vi "7_Hole_Probe Pressures to UVW_All_Ps.vi"() -> ()   [LabVIEW 2017]
uses:
  Controls/Setup.ctl
  Globals/Meas_global.vi
panel:
  in  "Desired Freq Hz":dbl=50.0
  out "Averaging samples":i32=5
  out "Current Case":string
  out "UVW chs":i32[](array[numeric])
  out "UVW":dbl[][](array[numeric])
  out "7 Hole Probe chs":string[](array[string])
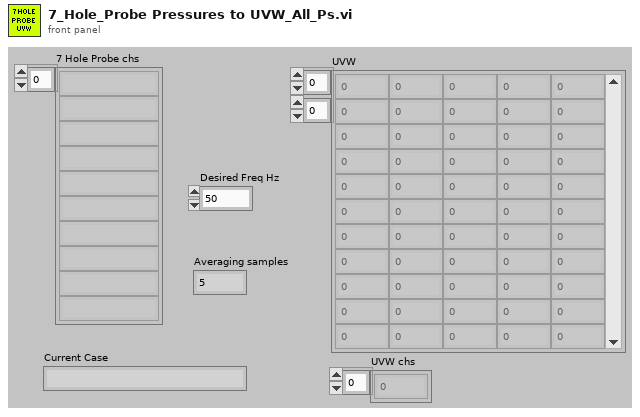
[diagram p1: front panel]
types:
  T1 = typedef "Analysis_info_cluster.ctl" = cluster{"Colour":u32, "Inst type":T2, "Inst name":string, "Symbol":string, "Code name":string, "Extra Info":string, "Inst Array":T3, "Extra Titles":string[], "Extra Values":string[], "U":dbl, "u^2":dbl, "u^3":dbl, "u^4":dbl, "Skew_u":dbl, "Kurt_u":dbl, "Sd Error in Mean":dbl, "% u'/U":dbl, "X":dbl, "Y":dbl, "Z":dbl, "Timescale integral Estimate":dbl, "Sd Error in Variance":dbl, "Calib File":path, "Calib Constants":dbl[], "Output Position":bool, "Full Stats":bool, "Av Sampling Rate":dbl, "Av No of Samples":dbl, "Total Meas Time (s)":dbl, "ADAM Ch Name":string, "Max value":dbl, "Min value":dbl, "Req Sample Rate Hz":dbl, "Sync Delay Time (s)":dbl, "Ch No":i16, "Device ID":string, "Use Latest Calib":bool, "Port":string}
  T2 = typedef "Inst_type.ctl" = enum16{"Propeller anemometer", "Raw voltage", "Pressure Transducer", "Pitot-static tube", "Preston tube", "Hot wire", "Cross wire 1", "Cross wire 2", "Generic Linear", "Generic Polynomial", "Generic BackPoly", "Fast FID", "Thermocouple", "Cold wire", "Pulsed Wire", "LDA Vel", "LDA Tran time", "LDA Arr time", "Microphone"}
  T3 = typedef "Instrument_Array.ctl" = enum16{"PWA", "LDA", "Analogue"}
  T4 = typedef "Time_Trace_Cluster.ctl" = cluster{"Weighting":dbl[], "Time (s)":dbl[], "Voltage":dbl[], "Eng Values":dbl[]}
  T5 = typedef "Setup.ctl" = enum16{"Run Program", "Show Setup", "Save Current Setup", "Setup Front Panel"}
  T6 = cluster{"Pressure Ch Names":string[], "Pressure Index":i32[], "Metadata Index":i32[], "Port":string}[]
  T7 = cluster{"Pressure Ch Names":string[], "Pressure Index":i32[], "Metadata Index":i32[], "Port":string}
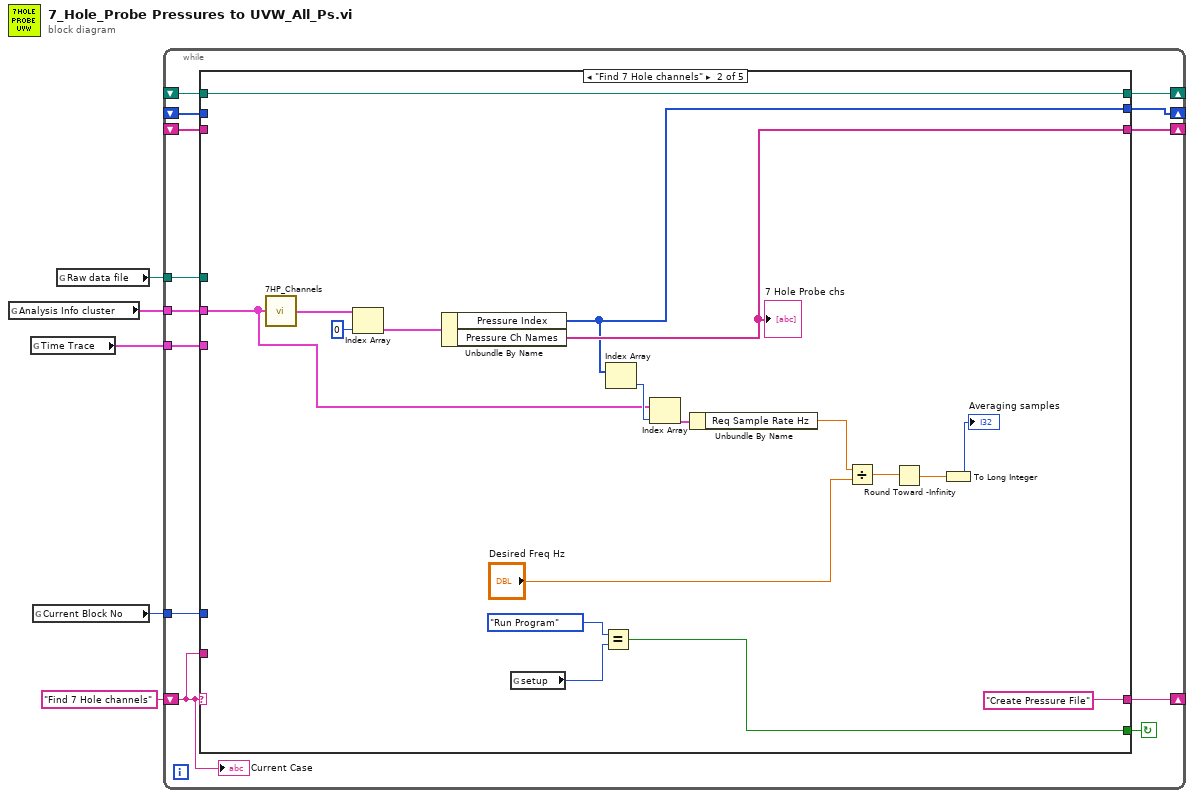
[diagram p0: block diagram]
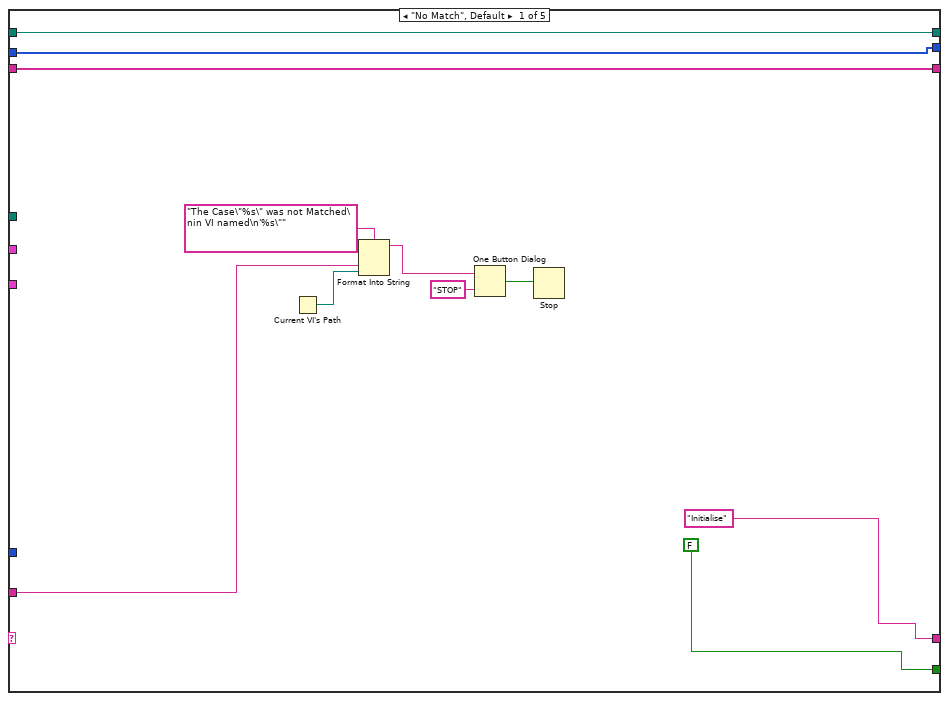
[diagram p2: hidden frame]
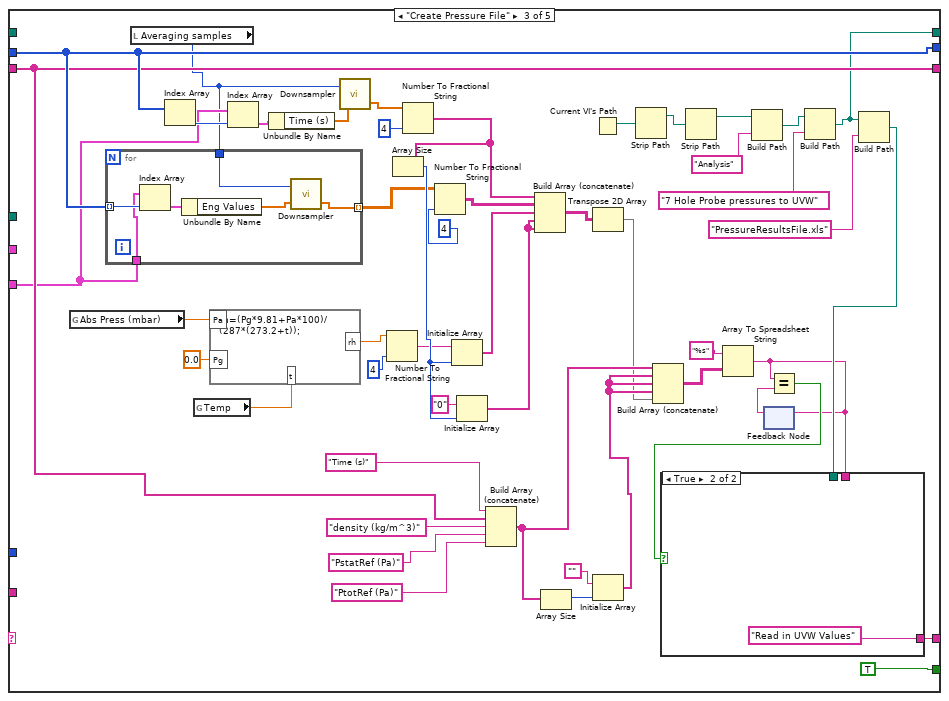
[diagram p3: hidden frame]
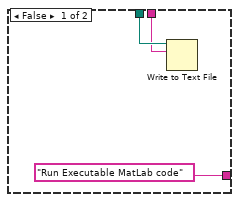
[diagram p4: hidden frame]
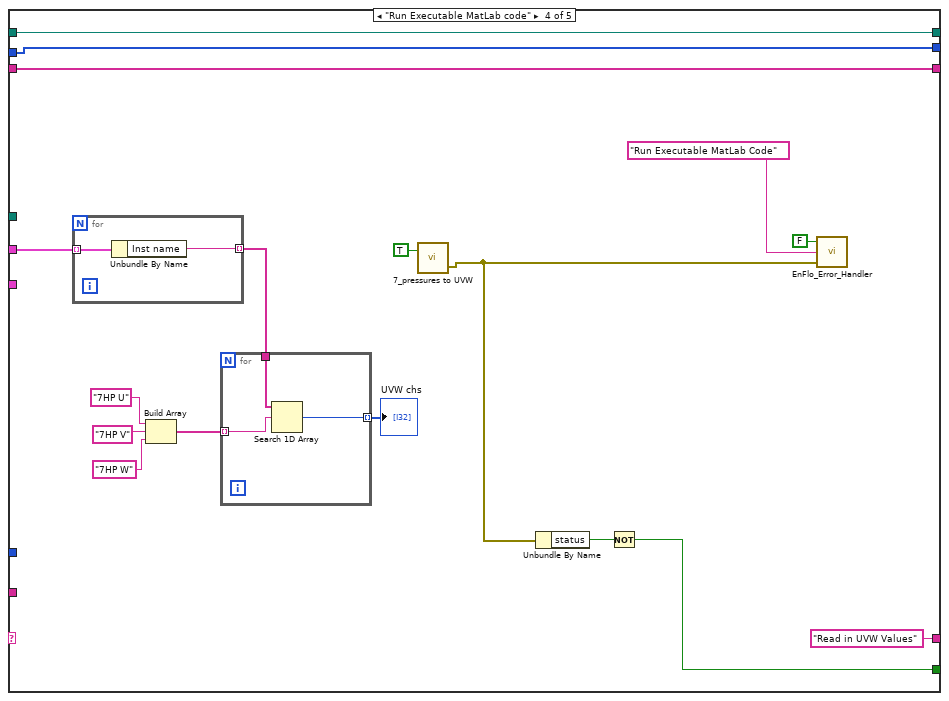
[diagram p5: hidden frame]
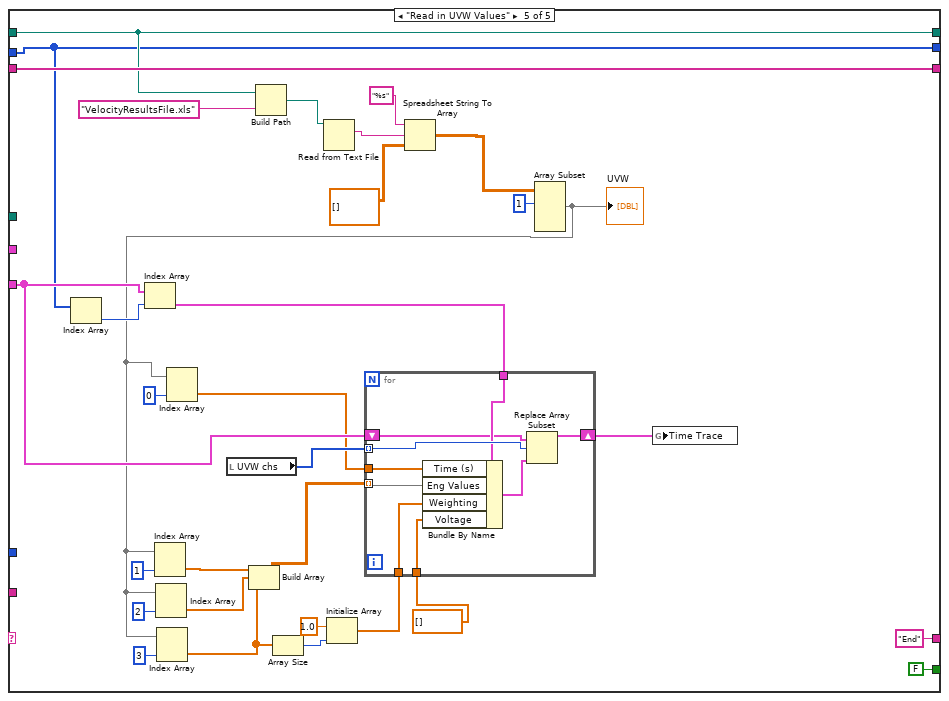
[diagram p6: hidden frame]
diagram:
  n1 = global read "Meas_global.vi" "Analysis Info cluster"() -> (w3:T1[])
  n2 = global read "Meas_global.vi" "Time Trace"() -> (w2:T4[])
  n3 = global read "Meas_global.vi" "Current Block No"() -> (w1:i32)
  n4 = global read "Meas_global.vi" "Raw data file"() -> (w4:path)
  n5 = while {
    shift-left: "Find 7 Hole channels" -> [w6]
    shift-right: [w7] -> _
    tunnel: w4 -> [w17]
    tunnel: w3 -> [w16]
    shift-right: [w15] -> _
    shift-left: _ -> [w14]
    shift-right: [w13] -> _
    shift-left: _ -> [w12]
    shift-right: [w11] -> _
    shift-left: _ -> [w10]
    tunnel: w2 -> [w9]
    tunnel: w1 -> [w8]
    stop <- w18 continue-if-true
    n6 = case shown="\"Find 7 Hole channels\"" w6 {
      tunnel: [FALSE w43 TRUE w107 FALSE] -> w18
      tunnel: ["Initialise" "Create Pressure File" ("t") w95 "Read in UVW Values" ("t") "End" ("t")] -> w7
      tunnel: w6 -> [w24 _ _ _ _]
      tunnel: w17 -> [_ _ _ _ _]
      tunnel: w16 -> [_ w36 _ w115 _]
      tunnel: [w21 w38 w94 w123 w139] -> w15
      tunnel: w14 -> [w21 _ w94 w123 w139]
      tunnel: [w20 w39 w69 w122 w159] -> w13
      tunnel: w12 -> [w20 _ w69 w122 w159]
      tunnel: [w19 w46 w55 w111 w156] -> w11
      tunnel: w10 -> [w19 w46 _ w111 w156]
      tunnel: w9 -> [_ _ w54 _ w140]
      tunnel: w8 -> [_ _ _ _ _]
      frame "No Match", Default {
        n7 = Current VI's Path() -> (path=w23:path)
        n8 = Format Into String(format string="The Case\"%s\" was not Matched\nin VI named\n'%s\"" ("Format String"), w24, w23) -> (resulting string=w27:string)  [unwired: 2 in, 1 out]
        n9 = One Button Dialog(message=w27, button name ("OK")="STOP") -> (true=w25:bool)
        n10 = Stop(stop? (T)=w25) -> ()
      }
      frame "Find 7 Hole channels" {
        n11 = call "7HP_Channels.vi"("Analysis Info cluster"=w36) -> ("7HP Info"=w42:T6)
        n12 = Index Array(array=w42, index=0 ("index (row)")) -> (element=w40:T7)
        n13 = Unbundle By Name(w40) -> ("Pressure Index"=w38:i32[], "Pressure Ch Names"=w39:string[])
        "7 Hole Probe chs" <- w39
        n14 = global read "Meas_global.vi" "setup"() -> (w45:T5)
        n15 = Equal?(x=Setup."Run Program" ("setup"), y=w45) -> (x = y?=w43:bool)
        n16 = Index Array(array=w38) -> (element=w37:i32)  [unwired: 1 in]
        n17 = Index Array(array=w36, index=w37) -> (element=w35:T1)
        n18 = Unbundle By Name(w35) -> ("Req Sample Rate Hz"=w34:dbl)
        n19 = Divide(x=w34, y="Desired Freq Hz") -> (x/y=w32:dbl)
        n20 = Round Toward -Infinity(1:w32) -> (0:w31:dbl)
        n21 = To Long Integer(number=w31) -> (32bit integer=→"Averaging samples":i32)
      }
      frame "Create Pressure File" {
        n22 = global read "Meas_global.vi" "Abs Press (mbar)"() -> (w90:dbl)
        n23 = local read "Averaging samples"() -> (w48:i32)
        n24 = for {
          tunnel: w94 -> [w106] mode=indexing
          tunnel: [w102] -> w77 mode=indexing
          tunnel: w54 -> [w104]
          tunnel: w48 -> [w101]
          n25 = Index Array(array=w104, index=w106) -> (element=w105:T4)
          n26 = Unbundle By Name(w105) -> ("Eng Values"=w103:dbl[])
          n27 = call "Downsampler.vi"("Input Array"=w103, "Averaging samples"=w101) -> ("Downsampled Array"=w102:dbl[])  [unwired: 1 out]
        }
        n28 = Index Array(array=w94) -> (element=w92:i32)  [unwired: 1 in]
        n29 = global read "Meas_global.vi" "Temp"() -> (w91:dbl)
        n30 = formula code="rh=(Pg*9.81+Pa*100)/\n(287*(273.2+t));"("t"=w91, "Pg"=0.0 ("input variable"), "Pa"=w90) -> ("rh"=w74:dbl)
        n31 = Index Array(array=w54, index=w92) -> (element=w93:T4)
        n32 = Unbundle By Name(w93) -> ("Time (s)"=w50:dbl[])
        n33 = call "Downsampler.vi"("Input Array"=w50, "Averaging samples"=w48) -> ("Downsampled Array"=w49:dbl[])  [unwired: 1 out]
        n34 = Number To Fractional String(number=w74, precision (6)=i16 4) -> (F-format string=w73:string)  [unwired: 2 in]
        n35 = Number To Fractional String(number=w49, precision (6)=i16 4) -> (F-format string=w79:string[])  [unwired: 2 in]
        n36 = Array Size(array=w79) -> (size(s)=w88:i32)
        n37 = Number To Fractional String(number=w77, precision (6)=i16 4) -> (F-format string=w76:string[][])  [unwired: 2 in]
        n38 = Initialize Array(w73, w88) -> (w86:string[])
        n39 = Initialize Array("0" ("element"), w88) -> (w85:string[])
        n40 = Build Array (concatenate)("Time (s)", w69, "density (kg/m^3)", "PstatRef (Pa)", "PtotRef (Pa)") -> (w60:string[])
        n41 = Build Array (concatenate)(w79, w76, w86, w85, w85) -> (w72:string[][])
        n42 = Array Size(array=w60) -> (size(s)=w59:i32)
        n43 = Current VI's Path() -> (path=w68:path)
        n44 = Transpose 2D Array(2D array=w72) -> (transposed array=w56:string[][])
        n45 = Initialize Array("", w59) -> (w57:string[])
        n46 = Strip Path(path=w68) -> (stripped path=w67:path)  [unwired: 1 out]
        n47 = Build Array (concatenate)(w60, w57, w57, w57, w56) -> (w71:string[][])
        n48 = Strip Path(path=w67) -> (stripped path=w66:path)  [unwired: 1 out]
        n49 = Array To Spreadsheet String(array=w71, 3:"%s" ("format string")) -> (spreadsheet string=w51:string)  [unwired: 1 in]
        n50 = Build Path(base path=w66, name or relative path="Analysis") -> (appended path=w64:path)
        n51 = feedback-in #1(w51) -> ()
        n52 = feedback #1() -> (w53:string)  [unwired: 1 in]
        n53 = Equal?(x=w51, y=w53) -> (x = y?=w52:bool)
        n54 = Build Path(base path=w64, name or relative path="7 Hole Probe pressures to UVW") -> (appended path=w55:path)
        n55 = Build Path(base path=w55, name or relative path="PressureResultsFile.xls") -> (appended path=w61:path)
        n56 = case shown="True" w52 {
          tunnel: ["Run Executable MatLab code" ("t") "Read in UVW Values" ("t")] -> w95
          tunnel: w61 -> [w99 _]
          tunnel: w51 -> [w98 _]
          frame False {
            n57 = Write to Text File(file (use dialog)=w99, text=w98) -> ()  [unwired: 2 in, 3 out]
          }
          frame True {
          }
        }
      }
      frame "Run Executable MatLab code" {
        n58 = for {
          tunnel: w115 -> [w128] mode=indexing
          tunnel: [w127] -> w114 mode=indexing
          n59 = Unbundle By Name(w128) -> ("Inst name"=w127:string)
        }
        n60 = Build Array("7HP U" ("Inst name"), "7HP V" ("Inst name"), "7HP W" ("Inst name")) -> (w113:string[])
        n61 = for {
          tunnel: w114 -> [w126]
          tunnel: w113 -> [w125] mode=indexing
          tunnel: [w124] -> w112 mode=indexing
          n62 = Search 1D Array(1D array=w126, element=w125) -> (index of element=w124:i32)  [unwired: 1 in]
        }
        "UVW chs" <- w112
        n63 = call "7_pressures to UVW.vi"("wait until completion?"=TRUE) -> ("error out"=w109:errorcluster)  [unwired: 2 in]
        n64 = Unbundle By Name(w109) -> ("status"=w108:bool)
        n65 = Not(x=w108) -> (.not. x?=w107:bool)
        n66 = call "EnFlo_Error_Handler.vi"("error in (no error)"=w109, "Error Type"="Run Executable MatLab Code", "Dialog Box (T)"=FALSE) -> ()  [unwired: 3 out]
      }
      frame "Read in UVW Values" {
        n67 = Index Array(array=w139) -> (element=w138:i32)  [unwired: 1 in]
        n68 = Index Array(array=w140, index=w138) -> (element=w137:T4)
        n69 = local read "UVW chs"() -> (w141:i32[])
        n70 = Build Path(base path=w156, name or relative path="VelocityResultsFile.xls") -> (appended path=w154:path)
        n71 = Read from Text File(file (use dialog)=w154) -> (text=w153:string)  [unwired: 3 in, 3 out]
        n72 = Spreadsheet String To Array(format string="%s", spreadsheet string=w153, array type (2D Dbl)=dbl[][] []) -> (array=w150:dbl[][])  [unwired: 1 in]
        n73 = Array Subset(array=w150, index (row)=1 ("index")) -> (w135:dbl[][])  [unwired: 3 in]
        "UVW" <- w135
        n74 = Index Array(array=w135, index (col)=1 ("disabled index (col)")) -> (element=w145:dbl[])  [unwired: 1 in]
        n75 = Index Array(array=w135, index (col)=2 ("disabled index (col)")) -> (element=w144:dbl[])  [unwired: 1 in]
        n76 = Index Array(array=w135, index (col)=3 ("disabled index (col)")) -> (element=w133:dbl[])  [unwired: 1 in]
        n77 = Index Array(array=w135, index (col)=0 ("disabled index (col)")) -> (element=w134:dbl[])  [unwired: 1 in]
        n78 = Build Array(w145, w144, w133) -> (w142:dbl[][])
        n79 = Array Size(array=w133) -> (size(s)=w132:i32)
        n80 = Initialize Array(1.0 ("element"), w132) -> (w130:dbl[])
        n81 = for {
          tunnel: w141 -> [w168] mode=indexing
          shift-right: [w167] -> w143
          shift-left: w140 -> [w163]
          tunnel: w142 -> [w166] mode=indexing
          tunnel: w137 -> [w164]
          tunnel: w134 -> [w162]
          tunnel: w130 -> [w161]
          tunnel: dbl[] [] ("Voltage") -> [w160]
          n82 = Bundle By Name(cluster=w164, "Time (s)"=w162, "Eng Values"=w166, "Weighting"=w161, "Voltage"=w160) -> (w165:T4)
          n83 = Replace Array Subset(array=w163, new element=w165, index=w168) -> (w167:T4[])
        }
        n84 = global write "Meas_global.vi" "Time Trace"(w143) -> ()
      }
    }
    "Current Case" <- w6
  }
